vi "MD5 Unrecoverable character padding.vi"(3 "Block Size (16)":i32=16, 5 "Message":string) -> (2 "Padded message":string)   [LabVIEW 2020]
doc: "Insert a number of <B>Padding Character</B> until the length of the string is a multiple of <B>Block Size</B>."
panel:
  # "[OpenG VI Tags] ***Do Not Remove***"
  # "MD5 Unrecoverable character padding.vi\n\nDerived from the RSA Data Security, Inc. MD5 Message-Digest Algorithm\n\nPlease visit http://www.OpenG.org to learn about the\nOpen Source LabVIEW software movement.\n\nNOTICE -- YOU MUST LEAVE THIS NOTICE IN PLACE.  PER THE TERMS OF THE LICENSE BELOW, YOU MAY SUBLICENSE THIS SOFTWARE \nIN ANY WAY THAT DOES NOT CONFLICT WITH THIS LICENSE.\n\n### BSD License (http://www.opensource.org/licenses/bsd-license.php) Begin ###\n \nCopyright (c) 2004, Enrique Vargas <vargas@visecurity.com>\n\nAll rights reserved.\n\nRedistribution and use in source and binary forms, with or without modification, are permitted provided that the following conditions are met:\n\n    * Redistributions of source code must retain the above copyright notice, this list of conditions and the following disclaimer.\n    * Redistributions in binary form must reproduce the above copyright notice, this list of conditions and the following disclaimer in the \n       documentation and/or other materials provided with the distribution.\n    * Neither the name of SciWare, James Kring, Inc., nor the names of its contributors may be used to endorse or promote products derived \n       from this software without specific prior written permission.\n\nTHIS SOFTWARE IS PROVIDED BY THE COPYRIGHT HOLDERS AND CONTRIBUTORS \"AS IS\" AND ANY EXPRESS OR IMPLIED WARRANTIES, \nINCLUDING, BUT NOT LIMITED TO, THE IMPLIED WARRANTIES OF MERCHANTABILITY AND FITNESS FOR A PARTICULAR PURPOSE ARE \nDISCLAIMED. IN NO EVENT SHALL THE COPYRIGHT OWNER OR CONTRIBUTORS BE LIABLE FOR ANY DIRECT, INDIRECT, INCIDENTAL,\n SPECIAL, EXEMPLARY, OR CONSEQUENTIAL DAMAGES (INCLUDING, BUT NOT LIMITED TO, PROCUREMENT OF SUBSTITUTE GOODS OR \nSERVICES; LOSS OF USE, DATA, OR PROFITS; OR BUSINESS INTERRUPTION) HOWEVER CAUSED AND ON ANY THEORY OF LIABILITY, \nWHETHER IN CONTRACT, STRICT LIABILITY, OR TORT (INCLUDING NEGLIGENCE OR OTHERWISE) ARISING IN ANY WAY OUT OF THE USE \nOF THIS SOFTWARE, EVEN IF ADVISED OF THE POSSIBILITY OF SUCH DAMAGE.\n\n### BSD License End ###"
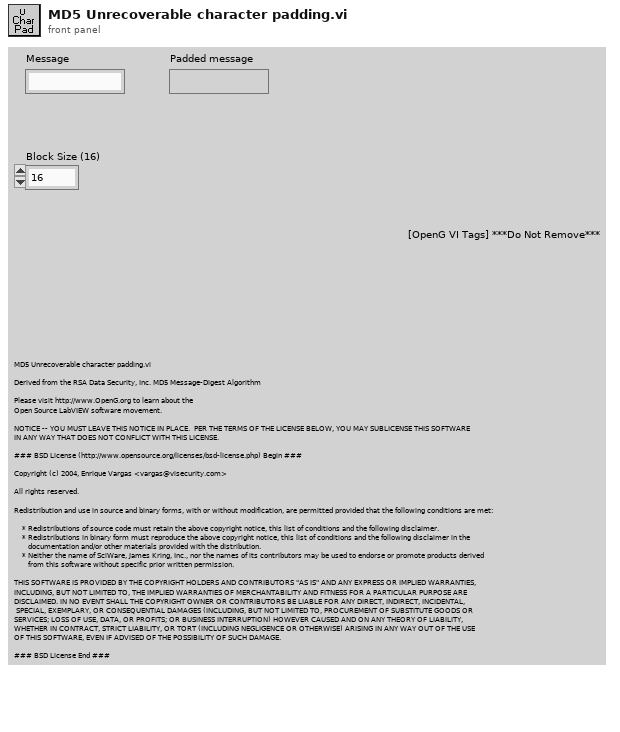
[diagram p1: front panel]
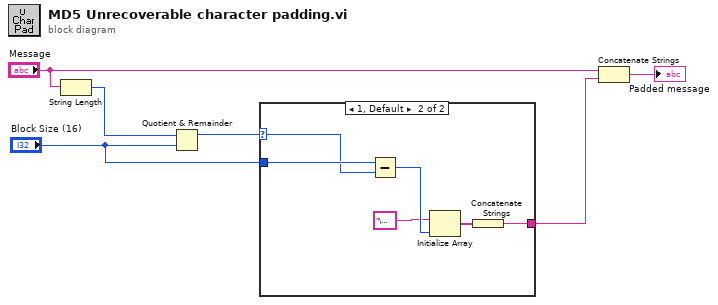
[diagram p0: block diagram]
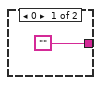
[diagram p2: hidden frame]
diagram:
  n1 = String Length(string="Message") -> (length=w1:i32)
  n2 = Quotient & Remainder(x=w1, y="Block Size (16)") -> (x-y*floor(x/y)=w2:i32)  [unwired: 1 out]
  n3 = case shown="1, Default" w2 {
    selector: w2 -> [_ w9]
    tunnel: "Block Size (16)" -> [_ w12]
    tunnel: ["" w10] -> w4
    frame 0 {
    }
    frame 1, Default {
      n4 = Subtract(x=w12, y=w9) -> (x-y=w11:i32)
      n5 = Initialize Array("\u0000" ("Padding Character (0)"), w11) -> (w13:string[])
      n6 = Concatenate Strings(w13) -> (w10:string)
    }
  }
  n7 = Concatenate Strings("Message", w4) -> (→"Padded message":string)
